vi "Global - Data.vi"() -> ()   [LabVIEW 2019, in "OWEN HMI.lvclass"]
uses:
  OWEN HMI.lvclass
panel:
  in  "SO":bool
  in  "CC":bool
  out "CHAMBER":bool
  out "DUT":bool
  in  "WARNING":bool
  in  "ALARM":bool
  in  "TEMP SO":i16
  in  "LEVEL SO":i16
  in  "TEMP CC":i16
  in  "LEVEL CC":i16
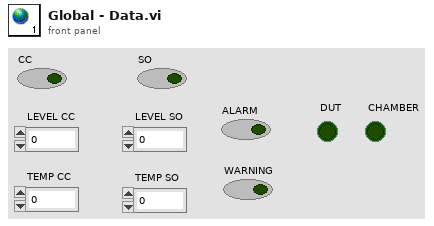
[diagram p1: front panel]
diagram:
